vi "Write Container Enqueuer.vi"(8 "error in (no error)":errorcluster, 10 "Actor Framework:Message Enqueuer":refnum<class "Message Enqueuer.lvclass">, 11 "GUI View in":refnum<class "GUI View.lvclass">) -> (0 "error out":errorcluster, 3 "GUI View out":refnum<class "GUI View.lvclass">)   [LabVIEW 2023, in "GUI Views.lvlib" / "GUI View.lvclass"]
uses:
  GUI View.lvclass
  <vilib>/ActorFramework/Message Enqueuer/Message Enqueuer.lvclass
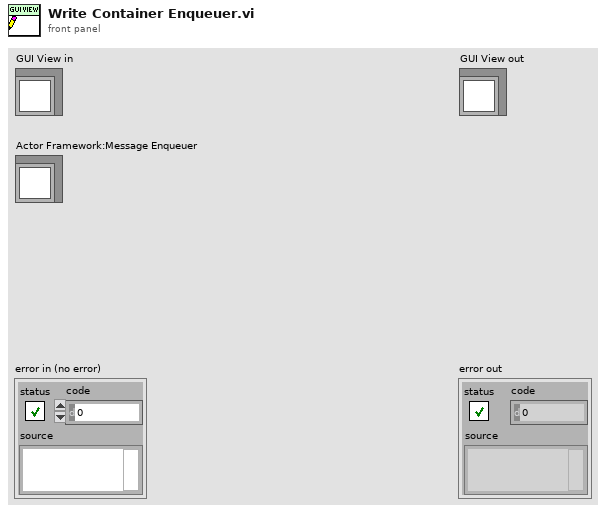
[diagram p1: front panel]
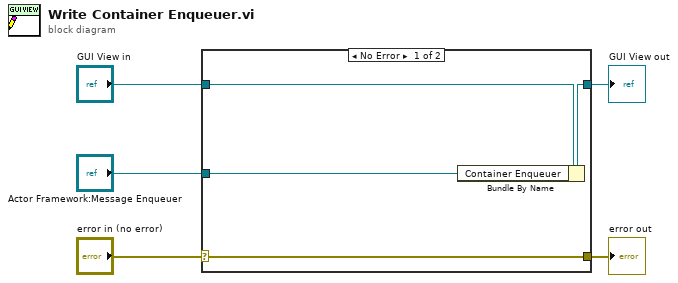
[diagram p0: block diagram]
diagram:
  n1 = case shown="No Error" "error in (no error)" {
    selector: "error in (no error)" -> [w9 w10]
    tunnel: [w9 w10] -> w4
    tunnel: [w7 w11] -> w2
    tunnel: "GUI View in" -> [w8 w11]
    tunnel: "Actor Framework:Message Enqueuer" -> [w6 _]
    frame No Error {
      n2 = Bundle By Name(cluster=w8, "Container Enqueuer"=w6) -> (w7:refnum<class "GUI View.lvclass">)
    }
    frame Error {
    }
  }
  "error out" <- w4
  "GUI View out" <- w2
